vi "Test Voltage Measurement Parsed when Measuring Voltage.vi"(8 "error in (no error)":errorcluster, 11 "Test Case In":refnum<class "Low Level PSU Test.lvclass">) -> (0 "error out":errorcluster, 3 "Test Case Out":refnum<class "Low Level PSU Test.lvclass">)   [LabVIEW 2020, in "Low Level PSU With Tests.lvlib" / "Low Level PSU Test.lvclass"]
uses:
  Low Level PSU Test.lvclass
  Low Level PSU Test.lvclass/Low Level PSU Test.ctl
  01074fa8-ee8a-411d-bc8b-fc92c4f90959.vi
  Mock Instrument Interface/Mock Instrument Interface.lvclass
  Low Level PSU/Low Level PSU.lvclass
  C:/Git/astemes-gdevcon-2022/PSU Demo/Low Level PSU With Tests/Mock Instrument Interface/Mock Instrument Interface.lvclass
  C:/Git/astemes-gdevcon-2022/PSU Demo/Instrument Interface/Instrument Interface.lvclass
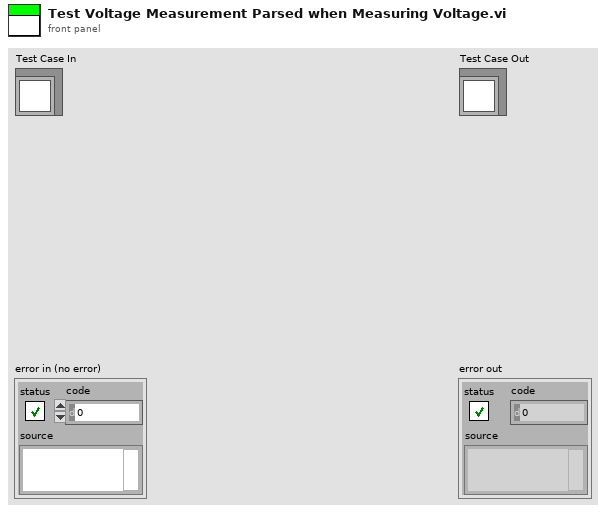
[diagram p1: front panel]
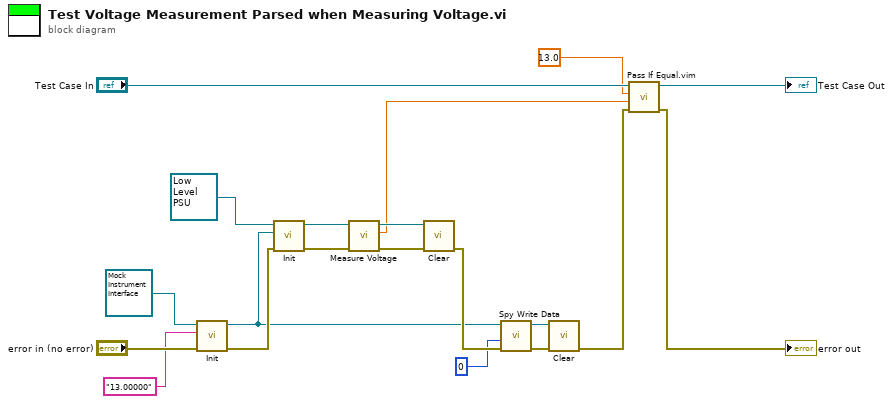
[diagram p0: block diagram]
diagram:
  n1 = call "Init.vi"("error in (no error)"="error in (no error)", "Response"="13.00000", "Mock Instrument Interface In"=refnum<class "Mock Instrument Interface.lvclass"> refnum) -> ("error out"=w13:errorcluster, "Mock Instrument Interface Out"=w6:refnum<class "Mock Instrument Interface.lvclass">)  [unwired: 7 in]
  n2 = call "Init.vi"("error in (no error)"=w13, "Instrument Interface"=w6, "Low Level PSU In"=refnum<class "Low Level PSU.lvclass"> refnum) -> ("error out"=w14:errorcluster, "Low Level PSU Out"=w15:refnum<class "Low Level PSU.lvclass">)  [unwired: 7 in]
  n3 = call "Measure Voltage.vi"("error in (no error)"=w14, "Low Level PSU In"=w15) -> ("error out"=w10:errorcluster, "Output Voltage"=w2:dbl, "Low Level PSU Out"=w11:refnum<class "Low Level PSU.lvclass">)  [unwired: 7 in]
  n4 = call "Clear.vi"("error in (no error)"=w10, "Low Level PSU In"=w11) -> ("error out"=w7:errorcluster)  [unwired: 8 in, 1 out]
  n5 = call "Spy Write Data.vi"("error in (no error)"=w7, "timeout in ms (-1)"=0, "Mock Instrument Interface in"=w6) -> ("error out"=w8:errorcluster, "Mock Instrument Interface out"=w9:refnum<class "Mock Instrument Interface.lvclass">)  [unwired: 5 in, 2 out]
  n6 = call "Clear.vi"("error in (no error)"=w8, "Mock Instrument Interface In"=w9) -> ("error out"=w4:errorcluster)  [unwired: 8 in, 1 out]
  n7 = call "Pass If Equal.vim"("error in (no error)"=w4, "Actual"=w2, "Expected"=13.0 ("Output Voltage"), "LUnit Test Case In"="Test Case In") -> ("error out"=→"error out":errorcluster, "LUnit Test Case Out"=→"Test Case Out":refnum<class "Low Level PSU Test.lvclass">)  [unwired: 6 in]
